vi "CloseSessions.vi"(8 "Motor IN":refnum<visa-resource-name>, 9 "Relay In":refnum<visa-resource-name>, 11 "Sessions In":T2) -> ()   [LabVIEW 2011]
uses:
  <vilib>/vision/Image Controls.llb/IMAQ Image.ctl
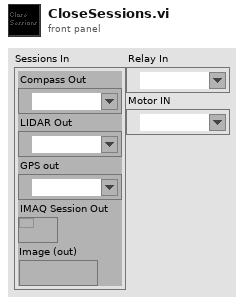
[diagram p1: front panel]
types:
  T1 = typedef "IMAQ Image.ctl" = refnum<image>
  T2 = cluster{"Compass Out":refnum<visa-resource-name>, "LIDAR Out":refnum<visa-resource-name>, "GPS out":refnum<visa-resource-name>, "IMAQ Session Out":refnum<k11>, "Image (out)":T1}
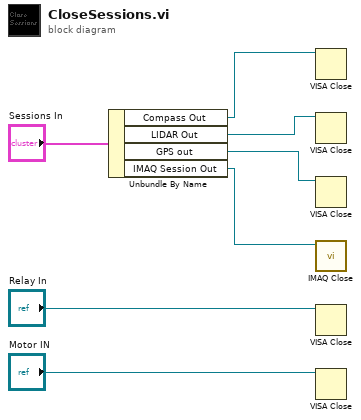
[diagram p0: block diagram]
diagram:
  n1 = Unbundle By Name("Sessions In") -> ("Compass Out"=w6:refnum<visa-resource-name>, "LIDAR Out"=w5:refnum<visa-resource-name>, "GPS out"=w4:refnum<visa-resource-name>, "IMAQ Session Out"=w3:refnum<k11>)
  n2 = VISA Close(VISA resource name=w6) -> ()  [unwired: 1 in, 1 out]
  n3 = VISA Close(VISA resource name=w5) -> ()  [unwired: 1 in, 1 out]
  n4 = VISA Close(VISA resource name=w4) -> ()  [unwired: 1 in, 1 out]
  n5 = call <vilib>:"IMAQ Close.vi"("IMAQ Session In"=w3) -> ()  [unwired: 10 in, 1 out]
  n6 = VISA Close(VISA resource name="Relay In") -> ()  [unwired: 1 in, 1 out]
  n7 = VISA Close(VISA resource name="Motor IN") -> ()  [unwired: 1 in, 1 out]
